vi "Set Initialization Data - Pumps Worker.vi"(8 "error in":errorcluster, 11 "gui in":refnum<class "gui.lvclass">) -> (0 "error out":errorcluster, 3 "gui out":refnum<class "gui.lvclass">)   [LabVIEW 2023, in "GUI.lvlib" / "gui.lvclass"]
doc: "In this VI you can set the initialization data of a statically-linked subWorker."
uses:
  gui.lvclass
  Pump_lvlib/Pumps Worker/Initialization Data.ctl
  Pump_lvlib/Pumps Worker/Response Cases.ctl
  <vilib>/addons/_Workers/Library/Case Label.ctl
  gui.lvclass/gui.ctl
  Pump_lvlib/Pumps Worker/Pumps Worker.lvclass
  C:/Program Files/National Instruments/LabVIEW 2023/vi.lib/addons/_Workers/Library/Classes/Worker/Worker.lvclass
  <vilib>/addons/_Workers/Library/Workers.lvlib
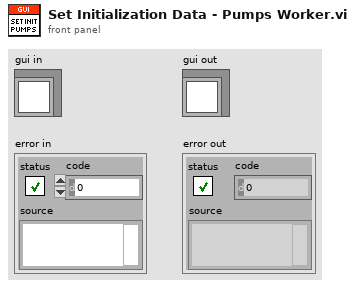
[diagram p1: front panel]
types:
  T1 = typedef "pump_Lib.lvlib/Pumps Worker.lvclass/Initialization Data.ctl" = cluster{"Response Cases":T2}
  T2 = typedef "pump_Lib.lvlib/Pumps Worker.lvclass/Response Cases.ctl" = cluster{"Placeholder - Can be deleted":string, "New Pumps Data":T3}
  T3 = typedef "Workers.lvlib/Case Label.ctl" = string
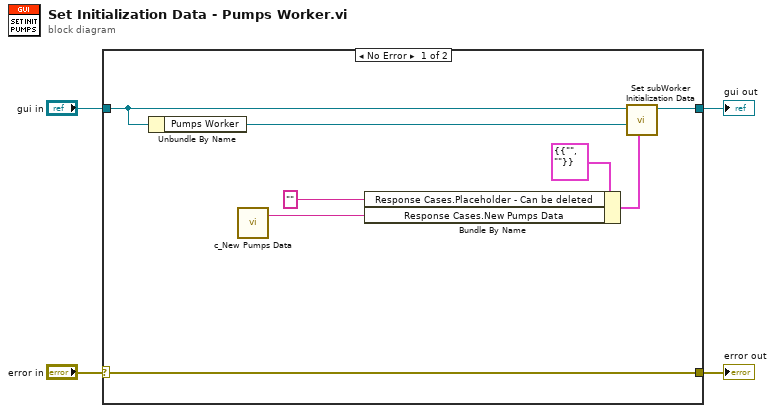
[diagram p0: block diagram]
diagram:
  n1 = case shown="No Error" "error in" {
    selector: "error in" -> [w12 w14]
    tunnel: [w12 w14] -> w3
    tunnel: [w10 w13] -> w2
    tunnel: "gui in" -> [w9 w13]
    frame No Error {
      n2 = Unbundle By Name(w9) -> ("Pumps Worker"=w11:refnum<class "Pumps Worker.lvclass">)
      n3 = call "c_New Pumps Data.vi"() -> ("Case Label"=w5:T3)  [unwired: 1 in]
      n4 = Bundle By Name(cluster=T1 {"Response Cases"={"Placeholder - Can be deleted"="", "New Pumps Data"=""}} ("Initialization Data"), "Response Cases.Placeholder - Can be deleted"="" ("Placeholder"), "Response Cases.New Pumps Data"=w5) -> (w7:T1)
      n5 = call-dynamic "Set subWorker Initialization Data.vi"("Initialization Data"=w7, "subWorker"=w11, "Worker"=w9) -> ("Worker out"=w10:refnum<class "gui.lvclass">)  [unwired: 8 in]
    }
    frame Error {
    }
  }
  "error out" <- w3
  "gui out" <- w2
